vi "tdms_dynmap.vi"() -> ()   [LabVIEW 2013]
uses:
  <vilib>/NI/Tag Bus Module Framework/channel/channel classification.ctl
  <vilib>/NI/Tag Bus Module Framework/runtime/execution settings.ctl
  TDMS datalogger/module/configuration/TDMS datalogger configuration.lvclass
  <vilib>/NI/Tag Bus/tag/Data Type.ctl
  TDMS datalogger/module/execution/TDMS datalogger runtime.lvclass
  <vilib>/NI/Tag Bus Module Framework/root configuration/TBM configuration.lvclass/TBM configuration.ctl
  TDMS datalogger/module/configuration/TDMS datalogger configuration.lvclass/TDMS datalogger configuration.ctl
  <vilib>/NI/Tag Bus/tag/tag descriptor.lvclass/tag descriptor.ctl
  <vilib>/NI/Tag Bus Module Framework/channel/TBM channel.lvclass/TBM channel.ctl
  <vilib>/NI/Tag Bus/tag/read data type.vi
  <vilib>/NI/Tag Bus/tag/read tag name.vi
  <vilib>/NI/Tag Bus Module Framework/channel/Read channel classification.vi
  <vilib>/NI/Tag Bus/table/data polymorphs/write one/write Double.vi
  <vilib>/NI/Tag Bus Module Framework/root configuration/Read instance name.vi
  TDMS datalogger/module/configuration/Write channel pattern matches.vi
  TDMS datalogger/module/configuration/Write Path.vi
  TDMS datalogger/module/configuration/Write queue size.vi
  TDMS datalogger/module/configuration/Write scans per write.vi
  TDMS datalogger/module/configuration/Write backup directory.vi
  TDMS datalogger/module/configuration/Write add enable channel.vi
  <vilib>/NI/Tag Bus Module Framework/root configuration/create GUID.vi
  <vilib>/NI/Tag Bus/dictionary/locate tag.vi
  <vilib>/NI/Tag Bus Module Framework/channel/TBM channel.lvclass
  <vilib>/NI/Tag Bus/tag/tag descriptor.lvclass
  <vilib>/NI/Tag Bus/table/data table.lvlib
  <vilib>/NI/Tag Bus/dictionary/data dictionary.lvclass
  <vilib>/NI/Tag Bus Module Framework/runtime/TBM module execution interface.lvclass
panel:
  in  "stop":bool
  out "error out":errorcluster
  out "execution settings":T1
  out "all classes":T2[](array[typedef])
  out "all names":string[](array[string])
  out "remote class":T2[](array[typedef])
  out "remote name":string[](array[string])
  out "local name":string[](array[string])
  out "local class":T2[](array[typedef])
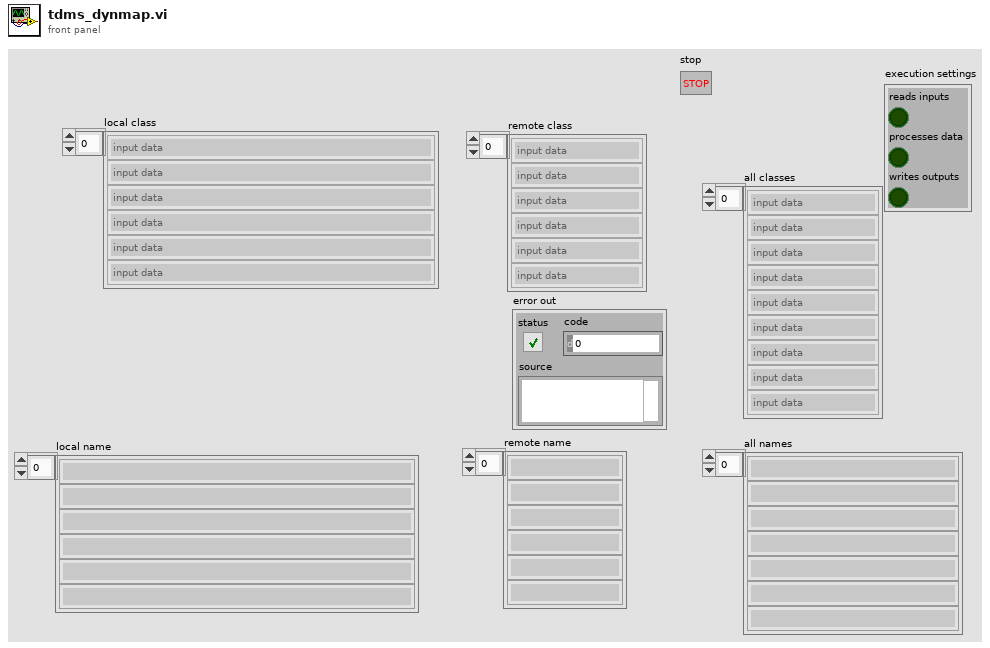
[diagram p1: front panel]
types:
  T1 = typedef "TBM module execution interface.lvclass/execution settings.ctl" = cluster{"reads inputs":bool, "processes data":bool, "writes outputs":bool}
  T2 = typedef "TBM channel.lvclass/channel classification.ctl" = enum16{"input data", "output data", "processing parameter", "processing result"}
  T3 = typedef "tag bus.lvlib/tag descriptor.lvclass/Data Type.ctl" = enum16{"Double", "Single", "I64", "I32", "I16", "I8", "U64", "U32", "U16", "U8", "Boolean", "String", "Array of Double", "Array of Single", "Array of I64", "Array of I32", "Array of I16", "Array of I8", "Array of U64", "Array of U32", "Array of U16", "Array of U8", "Array of Boolean", "Array of String"}
  T4 = typedef "TBM module configuration.lvclass/channel reservation.ctl" = cluster{"local channel":refnum<class "TBM channel.lvclass">, "remote channel":refnum<class "TBM channel.lvclass">}
  T5 = typedef "TBM channel.lvclass/data tables.ctl" = cluster{"input data":T6, "processing parameter":T6, "processing result":T6, "output data":T6}
  T6 = typedef "tag bus.lvlib/dictionary table pair.ctl" = cluster{"data dictionary":refnum<class "data dictionary.lvclass">, "data table":T7}
  T7 = typedef "tag bus.lvlib/data table.lvlib/data table.ctl" = cluster{"Double":dbl[], "Single":sgl[], "I64":i64[], "I32":i32[], "I16":i16[], "I8":i8[], "U64":u64[], "U32":u32[], "U16":u16[], "U8":u8[], "Boolean":bool[], "String":string[], "Array of Double":cluster{"DBL Array":dbl[]}[], "Array of Single":cluster{"SGL Array":sgl[]}[], "Array of I64":cluster{"I64 Array":i64[]}[], "Array of I32":cluster{"I32 Array":i32[]}[], "Array of I16":cluster{"I16 Array":i16[]}[], "Array of I8":cluster{"I8 Array":i8[]}[], "Array of U64":cluster{"U64 Array":u64[]}[], "Array of U32":cluster{"U32 Array":u32[]}[], "Array of U16":cluster{"U16 Array":u16[]}[], "Array of U8":cluster{"U8 Array":u8[]}[], "Array of Boolean":cluster{"Boolean Array":bool[]}[], "Array of String":cluster{"String Array":string[]}[]}
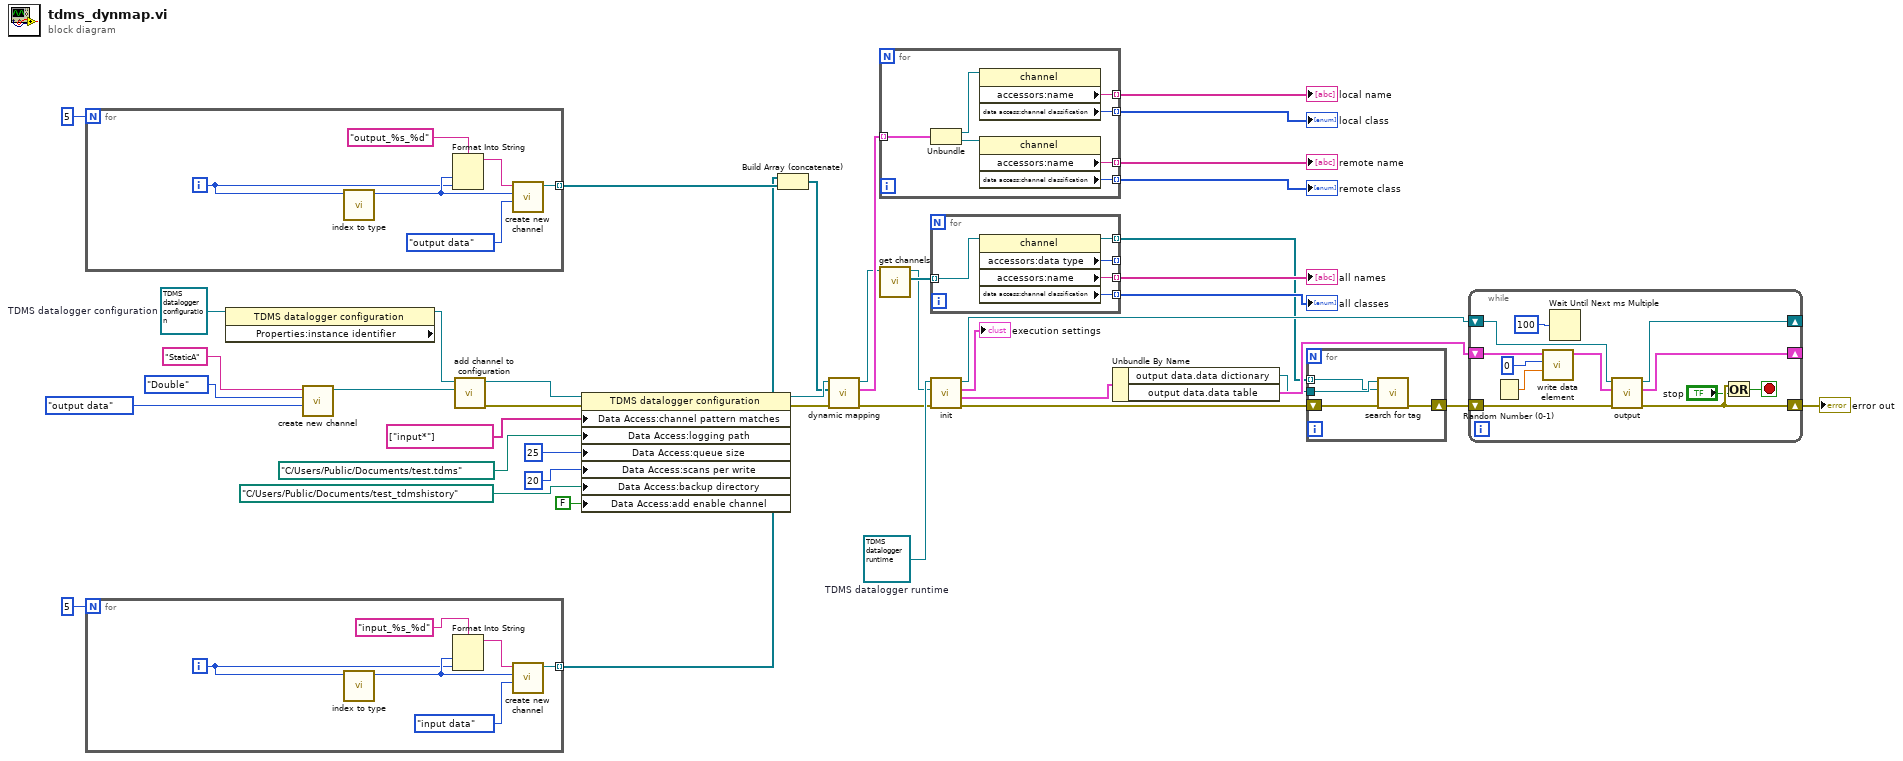
[diagram p0: block diagram]
diagram:
  w17 = refnum<class "TDMS datalogger runtime.lvclass"> refnum  # TDMS datalogger runtime
  w42 = refnum<class "TDMS datalogger configuration.lvclass"> refnum  # TDMS datalogger configuration
  n1 = for {
    N: 5 -> [_]
    tunnel: [w43] -> w35 mode=indexing
    i -> [w45]
    n2 = call <vilib>:"index to type.vi"("I32"=w45) -> ("type"=w47:T3)  [unwired: 10 in]
    n3 = Format Into String(format string="output_%s_%d", w47, w45) -> (resulting string=w44:string)  [unwired: 2 in, 1 out]
    n4 = call <vilib>:"create new channel.vi"("channel classification"=channel_classification."output data", "data type"=w47, "channel name"=w44) -> ("channel"=w43:refnum<class "TBM channel.lvclass">)  [unwired: 8 in]
  }
  n5 = for {
    N: 5 -> [_]
    tunnel: [w49] -> w34 mode=indexing
    i -> [w51]
    n6 = call <vilib>:"index to type.vi"("I32"=w51) -> ("type"=w53:T3)  [unwired: 10 in]
    n7 = Format Into String(format string="input_%s_%d", w53, w51) -> (resulting string=w50:string)  [unwired: 2 in, 1 out]
    n8 = call <vilib>:"create new channel.vi"("channel classification"=channel_classification."input data", "data type"=w53, "channel name"=w50) -> ("channel"=w49:refnum<class "TBM channel.lvclass">)  [unwired: 8 in]
  }
  n9 = property class="TDMS datalogger configuration" props=["Properties:instance identifier"](reference=w42) -> (reference out=w26:refnum<class "TDMS datalogger configuration.lvclass">)  [unwired: 1 in, 2 out]
  n10 = call <vilib>:"create new channel.vi"("channel classification"=channel_classification."output data", "data type"=Data_Type."Double", "channel name"="StaticA") -> ("channel"=w41:refnum<class "TBM channel.lvclass">)  [unwired: 8 in]
  n11 = call "add channel to configuration.vi"("TBM channel in"=w41, "TDMS datalogger configuration in"=w26) -> ("error out"=w33:errorcluster, "TDMS datalogger configuration out"=w31:refnum<class "TDMS datalogger configuration.lvclass">)  [unwired: 8 in]
  n12 = property class="TDMS datalogger configuration"(reference=w31, error in=w33, "Data Access:channel pattern matches"=string[] ["input*"] ("channel pattern matches"), "Data Access:logging path"=path "C:/Users/Public/Documents/test.tdms" ("logging path"), "Data Access:queue size"=25 ("queue size"), "Data Access:scans per write"=20 ("scans per write"), "Data Access:backup directory"=path "C:/Users/Public/Documents/test_tdmshistory" ("backup directory"), "Data Access:add enable channel"=FALSE ("add enable channel")) -> (reference out=w30:refnum<class "TDMS datalogger configuration.lvclass">, error out=w32:errorcluster)
  n13 = Build Array (concatenate)(w34, w35) -> (w28:refnum<class "TBM channel.lvclass">[])
  n14 = call-dynamic "dynamic mapping.vi"("error in"=w32, "channels available"=w28, "module configuration in"=w30) -> ("error out"=w15:errorcluster, "reservations"=w27:T4[], "module configuration out"=w21:refnum<class "TDMS datalogger configuration.lvclass">)  [unwired: 6 in]
  n15 = for {
    tunnel: w27 -> [w61] mode=indexing
    tunnel: [w59] -> w25 mode=indexing
    tunnel: [w58] -> w24 mode=indexing
    tunnel: [w56] -> w23 mode=indexing
    tunnel: [w55] -> w22 mode=indexing
    n16 = Unbundle(w61) -> ("local channel"=w60:refnum<class "TBM channel.lvclass">, "remote channel"=w57:refnum<class "TBM channel.lvclass">)
    n17 = property class="channel"(reference=w60) -> ("accessors:name"=w58:string, "data access:channel classification"=w59:T2)  [unwired: 1 in, 2 out]
    n18 = property class="channel"(reference=w57) -> ("accessors:name"=w56:string, "data access:channel classification"=w55:T2)  [unwired: 1 in, 2 out]
  }
  "local class" <- w25
  "local name" <- w24
  "remote class" <- w22
  "remote name" <- w23
  n19 = call-dynamic "get channels.vi"("module configuration in"=w21) -> ("channels"=w20:refnum<class "TBM channel.lvclass">[], "module configuration out"=w16:refnum<class "TDMS datalogger configuration.lvclass">)  [unwired: 9 in]
  n20 = for {
    tunnel: w20 -> [w66] mode=indexing
    tunnel: [w65] -> w19 mode=indexing
    tunnel: [w64] -> w18 mode=indexing
    tunnel: [w63] -> _ mode=indexing
    tunnel: [w62] -> w8 mode=indexing
    n21 = property class="channel"(reference=w66) -> (reference out=w62:refnum<class "TBM channel.lvclass">, "accessors:data type"=w63:T3, "accessors:name"=w65:string, "data access:channel classification"=w64:T2)  [unwired: 1 in, 1 out]
  }
  "all classes" <- w18
  "all names" <- w19
  n22 = call-dynamic "init.vi"("error in"=w15, "TBM module configuration in"=w16, "TDMS datalogger runtime in"=w17) -> ("error out"=w7:errorcluster, "data allocations"=w13:T5, "execution settings"=→"execution settings":T1, "TDMS datalogger runtime out"=w11:refnum<class "TDMS datalogger runtime.lvclass">)  [unwired: 5 in]
  n23 = Unbundle By Name(w13) -> ("output data.data dictionary"=w9:refnum<class "data dictionary.lvclass">, "output data.data table"=w12:T7)
  n24 = for {
    tunnel: w9 -> [w70]
    tunnel: w8 -> [w69] mode=indexing
    shift-right: [w68] -> w6
    shift-left: w7 -> [w67]
    n25 = call <vilib>:"search for tag.vi"("error in"=w67, "system tag"=w69, "data dictionary in"=w70) -> ("error out"=w68:errorcluster)  [unwired: 6 in, 2 out]
  }
  n26 = while {
    shift-right: [w77] -> _
    shift-left: w11 -> [w80]
    shift-right: [w76] -> _
    shift-left: w12 -> [w82]
    shift-right: [w74] -> w10
    shift-left: w6 -> [w73]
    stop <- w72 stop-if-true
    n27 = Random Number (0-1)() -> (number: 0 to 1=w79:dbl)
    n28 = call-poly <vilib>:"write data element.vi"("value"=w79, "index"=0, "data table in"=w82) -> ("data table out"=w75:T7)  [unwired: 8 in]
    n29 = Wait Until Next ms Multiple(millisecond multiple=u32 100) -> ()  [unwired: 1 out]
    n30 = call-dynamic "output.vi"("error in"=w73, "data table in"=w75, "TDMS datalogger runtime in"=w80) -> ("error out"=w74:errorcluster, "data table out"=w76:T7, "TDMS datalogger runtime out"=w77:refnum<class "TDMS datalogger runtime.lvclass">)  [unwired: 6 in]
    n31 = Or(x=w74, y="stop") -> (x .or. y?=w72:bool)
  }
  "error out" <- w10
